vi "Switchboard_main.vi"(8 "Error In":errorcluster) -> (0 "Error Out":errorcluster)   [LabVIEW 2013]
uses:
  My Computer/Controls/Steering Inputs.ctl
  My Computer/Controls/Intuitive Steering.ctl
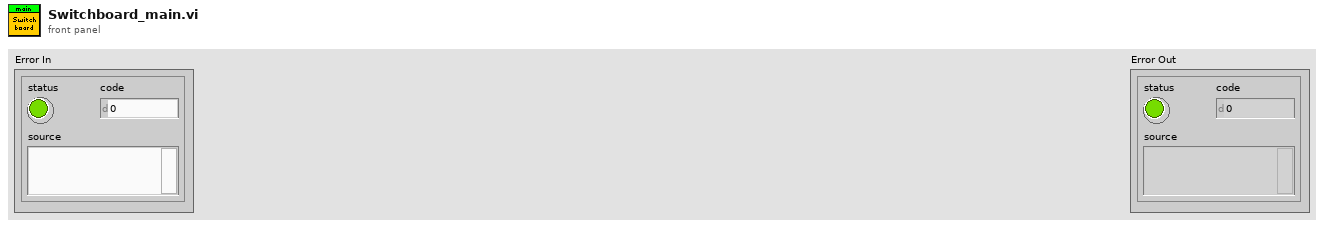
[diagram p1: front panel]
types:
  T1 = typedef "Steering Inputs.ctl" = cluster{"X":dbl, "Y":dbl, "Z":dbl, "phi":dbl, "theta":dbl, "psi":dbl}
  T2 = typedef "Intuitive Steering.ctl" = cluster{"Frequency (Hz):":dbl, "Max. Amplitude (°):":dbl, "Phase Shift (/Pi):":dbl, "Flap (°):":dbl, "Flap Saturation:":dbl}
  T3 = cluster{"X":dbl, "Y":dbl, "Z":dbl, "phi":dbl, "theta":dbl, "psi":dbl}
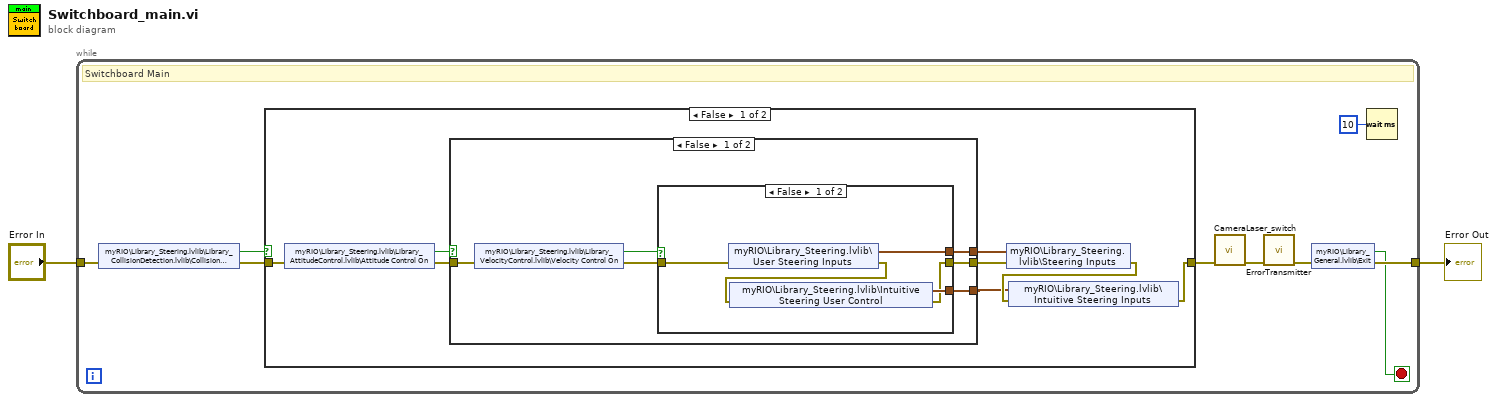
[diagram p0: block diagram]
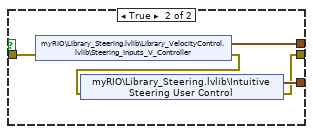
[diagram p2: hidden frame]
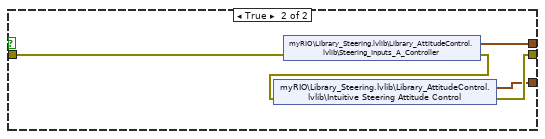
[diagram p3: hidden frame]
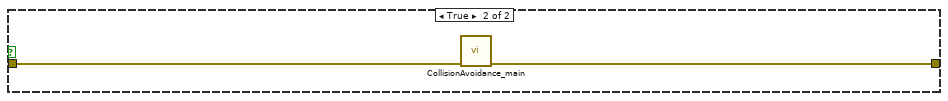
[diagram p4: hidden frame]
diagram:
  n1 = while {
    tunnel: "Error In" -> [w11]
    tunnel: [w10] -> w1
    stop <- w5 stop-if-true
    # "Switchboard Main"
    n2 = shared-variable "myRIO\\Library_Steering.lvlib\\Library_CollisionDetection.lvlib\\Collision Detected"(error in=w11) -> (w6:bool, error out=w7:errorcluster)
    n3 = case shown="False" w6 {
      tunnel: [w13 w41] -> w4
      tunnel: w7 -> [w17 w42]
      frame False {
        n4 = shared-variable "myRIO\\Library_Steering.lvlib\\Library_AttitudeControl.lvlib\\Attitude Control On"(error in=w17) -> (w16:bool, error out=w15:errorcluster)
        n5 = case shown="False" w16 {
          tunnel: [w25 w40] -> w19
          tunnel: w15 -> [w22 w39]
          tunnel: [w23 w37] -> w18
          tunnel: [w24 w36] -> w12
          frame False {
            n6 = shared-variable "myRIO\\Library_Steering.lvlib\\Library_VelocityControl.lvlib\\Velocity Control On"(error in=w22) -> (w20:bool, error out=w21:errorcluster)
            n7 = case shown="False" w20 {
              tunnel: [w30 w31] -> w25
              tunnel: w21 -> [w29 w33]
              tunnel: [w27 w35] -> w24
              tunnel: [w26 w34] -> w23
              frame False {
                n8 = shared-variable "myRIO\\Library_Steering.lvlib\\User Steering Inputs"(error in=w29) -> (w30:T1, error out=w28:errorcluster)
                n9 = shared-variable "myRIO\\Library_Steering.lvlib\\Intuitive Steering User Control"(error in=w28) -> (w27:T2, error out=w26:errorcluster)
              }
              frame True {
                n10 = shared-variable "myRIO\\Library_Steering.lvlib\\Library_VelocityControl.lvlib\\Steering_Inputs_V_Controller"(error in=w33) -> (w31:T3, error out=w32:errorcluster)
                n11 = shared-variable "myRIO\\Library_Steering.lvlib\\Intuitive Steering User Control"(error in=w32) -> (w35:T2, error out=w34:errorcluster)
              }
            }
          }
          frame True {
            n12 = shared-variable "myRIO\\Library_Steering.lvlib\\Library_AttitudeControl.lvlib\\Steering_Inputs_A_Controller"(error in=w39) -> (w40:T1, error out=w38:errorcluster)
            n13 = shared-variable "myRIO\\Library_Steering.lvlib\\Library_AttitudeControl.lvlib\\Intuitive Steering Attitude Control"(error in=w38) -> (w36:T2, error out=w37:errorcluster)
          }
        }
        n14 = shared-variable "myRIO\\Library_Steering.lvlib\\Steering Inputs"(w19, error in=w18) -> (error out=w14:errorcluster)
        n15 = shared-variable "myRIO\\Library_Steering.lvlib\\Intuitive Steering Inputs"(w12, error in=w14) -> (error out=w13:errorcluster)
      }
      frame True {
        n16 = call "CollisionAvoidance_main.vi"("Error In"=w42) -> ("Error Out"=w41:errorcluster)  [unwired: 10 in]
      }
    }
    n17 = call "CameraLaser_switch.vi"("error in (no error)"=w4) -> ("error out"=w3:errorcluster)  [unwired: 10 in]
    n18 = call "ErrorTransmitter.vi"("Error In"=w3) -> ("Error Out"=w8:errorcluster)  [unwired: 10 in]
    n19 = shared-variable "myRIO\\Library_General.lvlib\\Exit"(error in=w8) -> (w5:bool, error out=w10:errorcluster)
    n20 = Wait (ms)(milliseconds to wait=u32 10) -> ()  [unwired: 1 out]
  }
  "Error Out" <- w1
